vi "main 0.6.vi"() -> ()   [LabVIEW 2012]
uses:
  coherent/CH_LM/CH_LM Communication Mode.ctl
  ISEGNHQxxu/iseg NHQ VISA Control.ctl
  <vilib>/Utility/file.llb/Read From Spreadsheet File (DBL).vi
  <vilib>/Utility/file.llb/Write To Spreadsheet File (DBL).vi
  <vilib>/Analysis/1siggen.llb/Ramp Pattern by Samples.vi
  <vilib>/Analysis/NI_AALBase.lvlib
  coherent/CH_LM.lvlib
panel:
  out "laser power":sgl=6.5658234e-09 format="%^#_3e"
  out "Actual Voltage":dbl=-50.050000000000004 format="%.2f"
  out "Waveform Chart":dbl(graph)
  in  "Path":path=path "Y:/Ediff/data/2016/10/161018"
  in  "stop":bool
  out "Slide":dbl(slide)=0.999 scale=0.0..1.0
  in  "Tab Control":enum32{"live", "XY", "voltage scan", "settings"}(tab)
  in  "dark_load":bool
  in  "binning":dbl=4.0
  in  "exp time [s]":dbl=0.01
  in  "frames":i32=1000
  in  "avg[t] acc[f]":bool=TRUE
  in  "threshold":i32=110
  in  "dark?":bool=TRUE
  in  "dark":bool
  in  "snap":bool
  in  "count?":bool
  in  "save":bool
  in  "Nominal Voltage":sgl=50.0 max=4000 format="%.2f"
  in  "volt_set":bool
  in  "volt_threshold":sgl=2.0 max=4000 format="%.2f"
  in  "volt_timeout":u32=6000
  in  "move2com":bool
  in  "window2":dbl=10000.0 caption="+/- window" format="%#_6e"
  in  "steps2":u32=21 caption="steps"
  out "XY":dbl[][](graph)
  in  "meas_start_XY":bool
  in  "Axis2":string(combo)="4D Z"
  in  "Axis1":string(combo)="4D Z"
  in  "window1":dbl=10000.0 caption="+/- window" format="%#_6e"
  in  "steps1":u32=21 caption="steps"
  in  "meas_stop_XY":bool
  in  "showcom":bool
  out "XY Graph":cluster{"Ramp Pattern":dbl[], dbl[]}(graph)
  in  "voltage":string="225"
  in  "meas_stop_volt":bool
  in  "meas_start_vofalt":bool
  in  "head":string="PowerVoltScan1"
  in  "VISA ISEG":refnum<visa-resource-name>="COM6"
  in  "Channel (A)":enum16{"A", "B"}(ring)=enum."B"
  in  "IP address":string="172.24.192.135"
  out "error out":errorcluster
  out "coherent":errorcluster
  out "captured":dbl[][](graph)
  out "live":dbl[][](graph)
  in  "close":bool
  # "W"
  # "V"
  # "Axis2"
  # "Axis1"
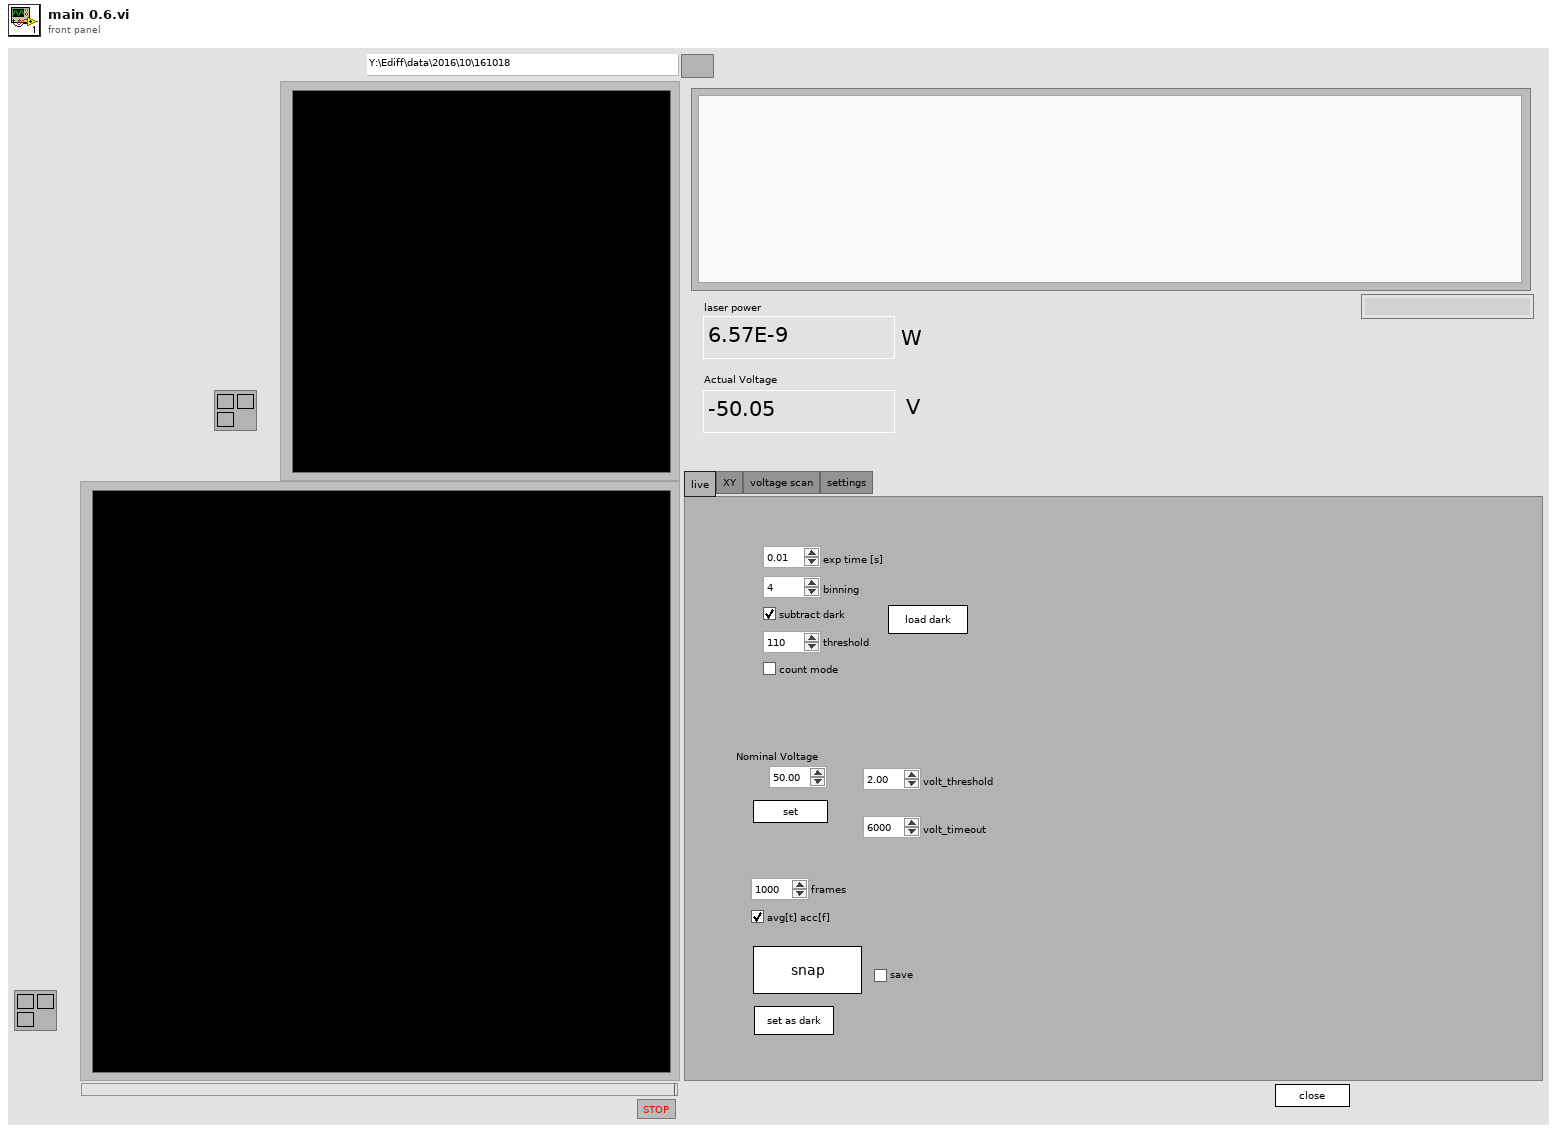
[diagram p1: front panel]
types:
  T1 = typedef "CH_LM.lvlib/CH_LM Communication Mode.ctl" = enum16{"None", "USB", "GPIB", "RS232"}
  T2 = cluster{"height":u32, "width":u32, "datatype":u32}
  T3 = typedef "iseg NHQ VISA Control.ctl" = cluster{"VISA Resource Name":refnum<visa-resource-name>, "FP Notation":bool, "Maximum Voltage":u32, "Maximum Current":u32}
  T4 = typedef "CH_LM.lvlib/CH_LM Streaming Data.ctl" = cluster{"Value":sgl, "Quad Distance":cluster{"X":sgl, "Y":sgl}, "Display Data":cluster{"Format ID":u8, "Scale ID":u8}, "Unit ID":u8, "Flags":u32, "Pulse Period":u32, "Sequence ID":u32, "Unit String":string}
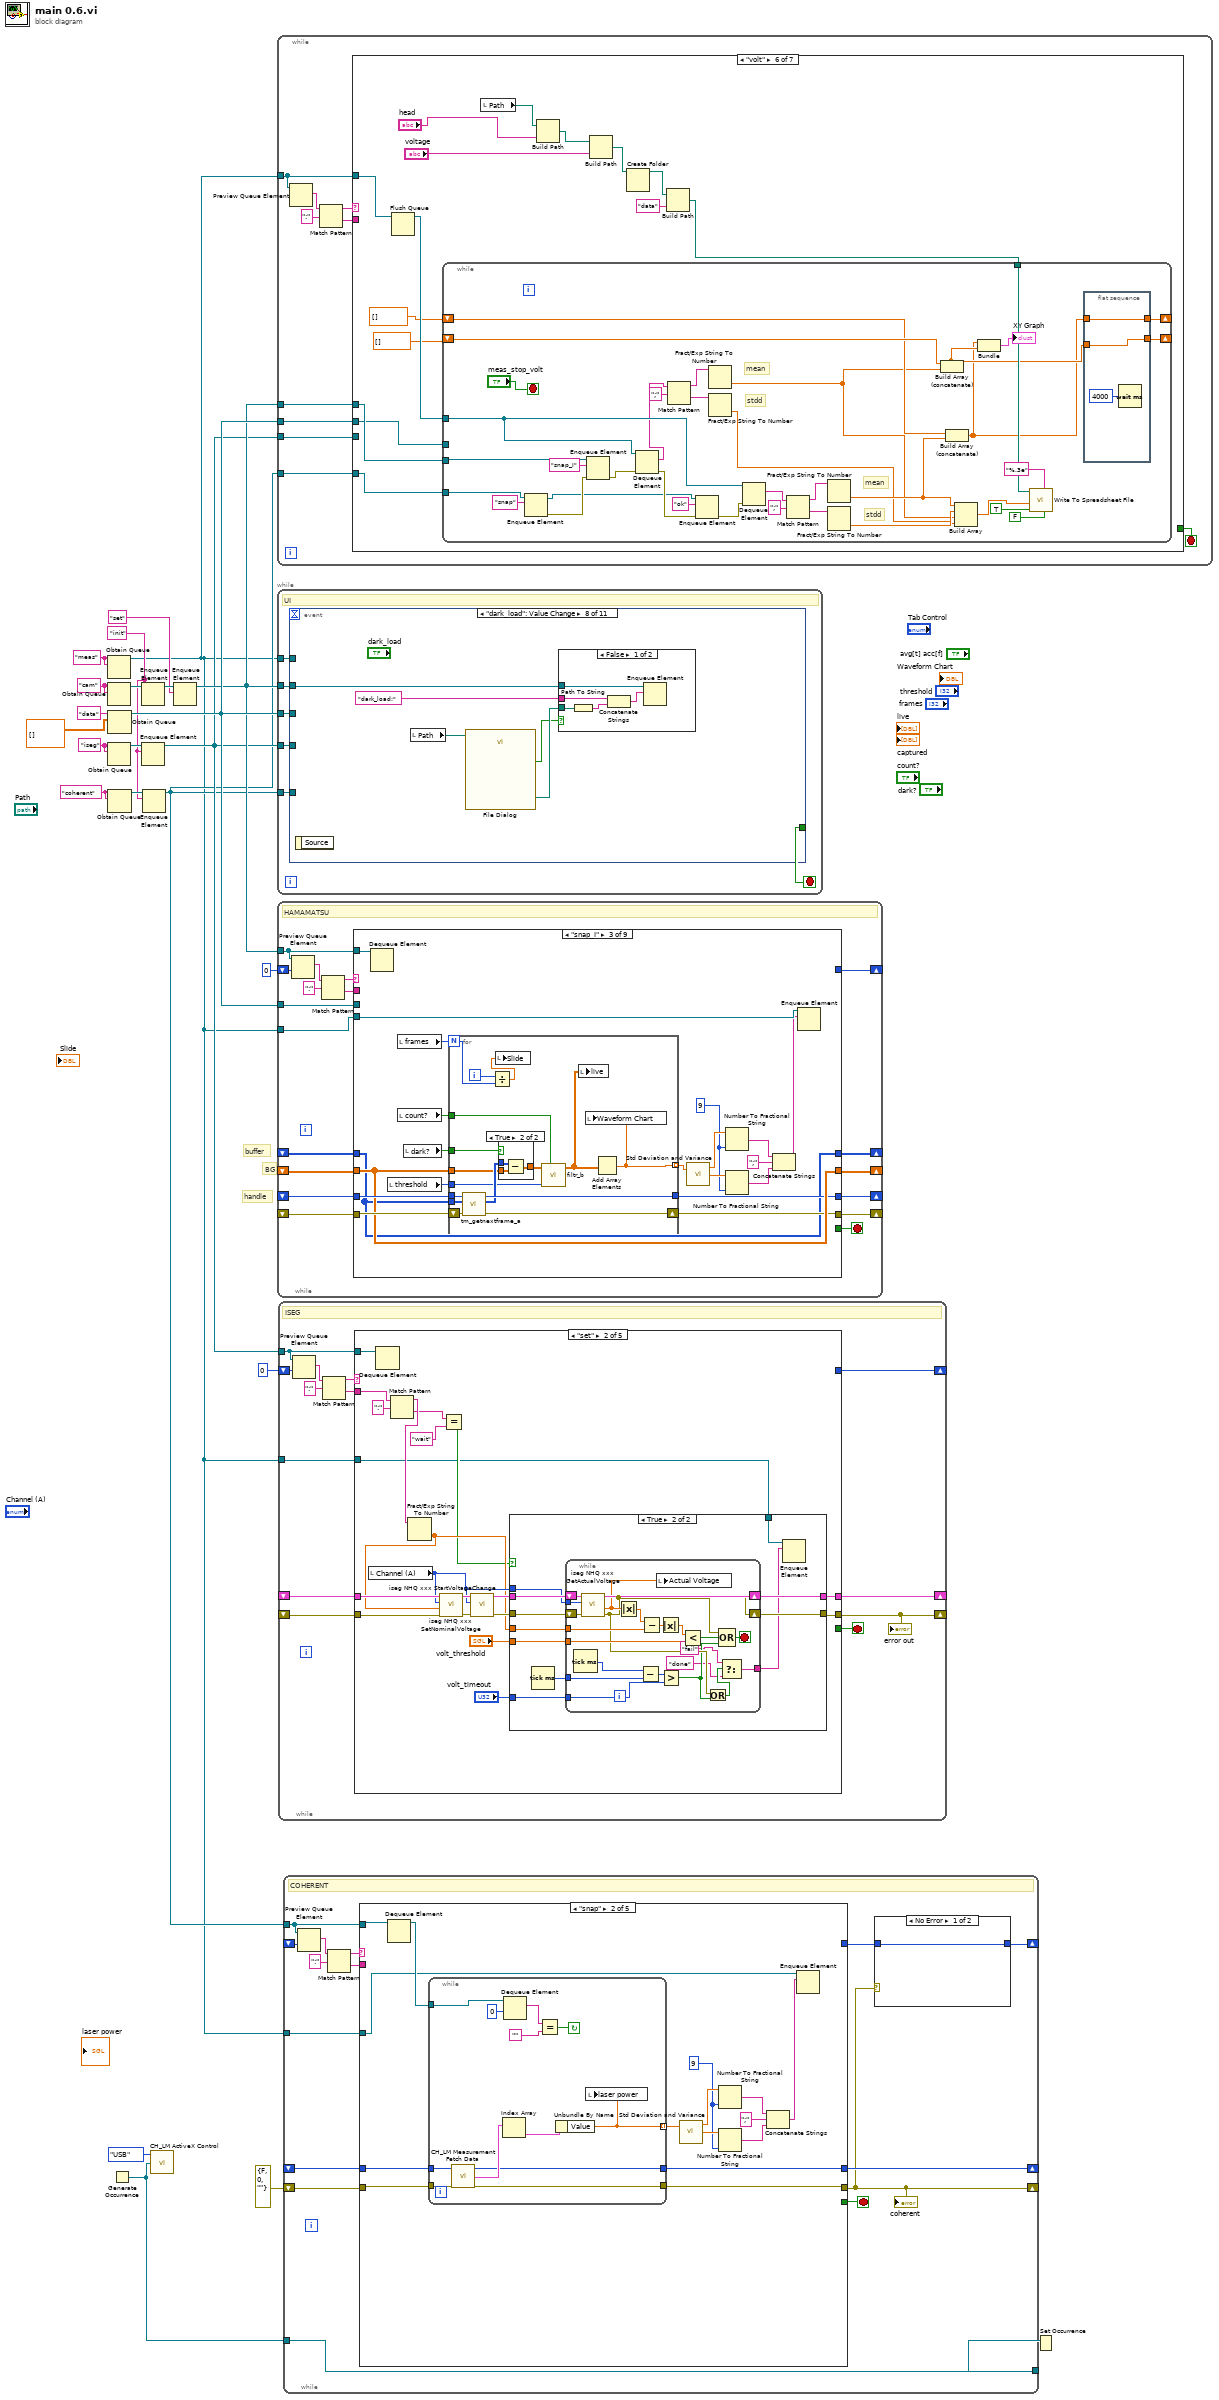
[diagram p0: block diagram]
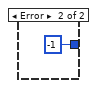
[diagram p2: hidden frame]
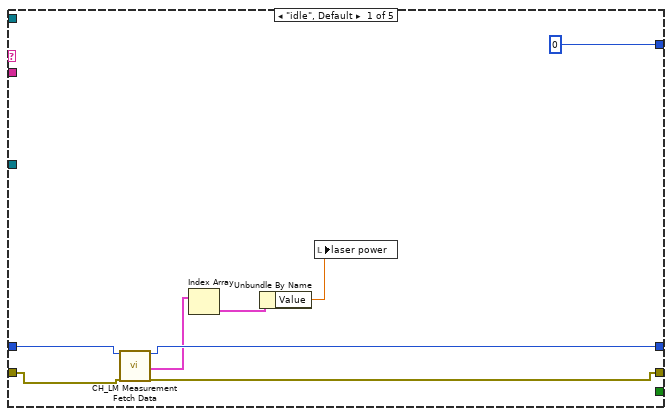
[diagram p3: hidden frame]
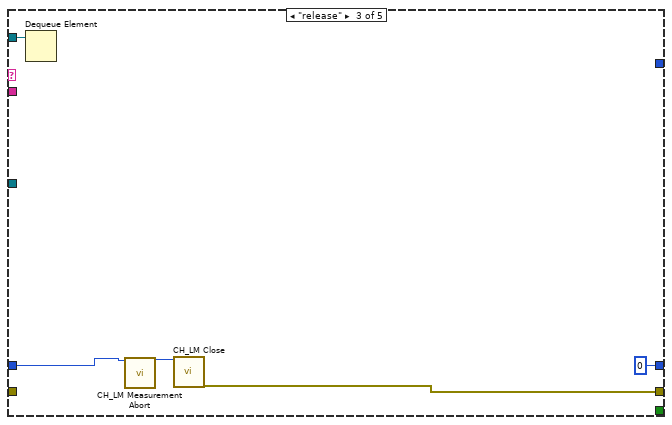
[diagram p4: hidden frame]
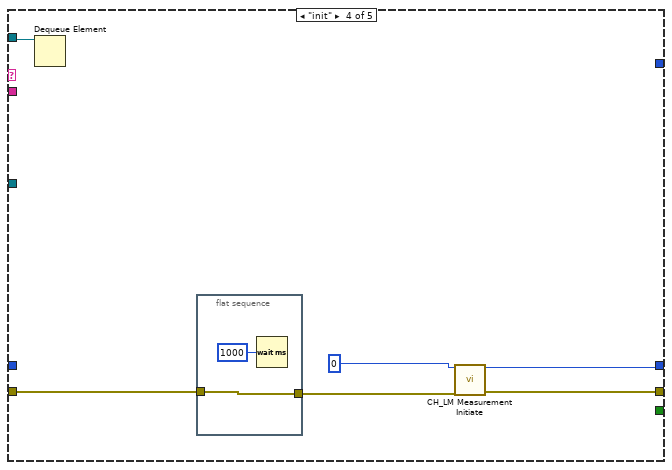
[diagram p5: hidden frame]
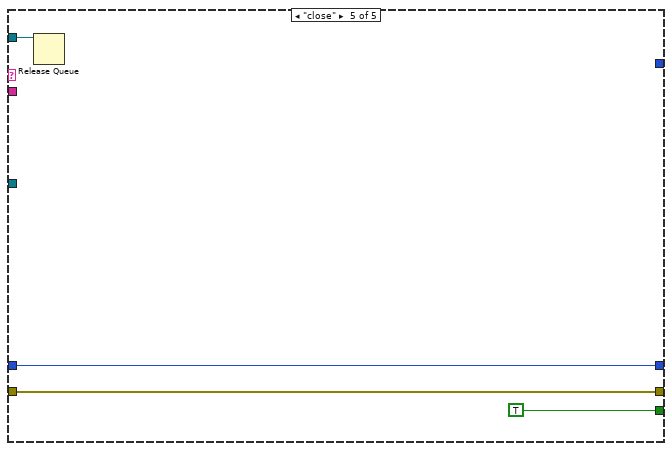
[diagram p6: hidden frame]
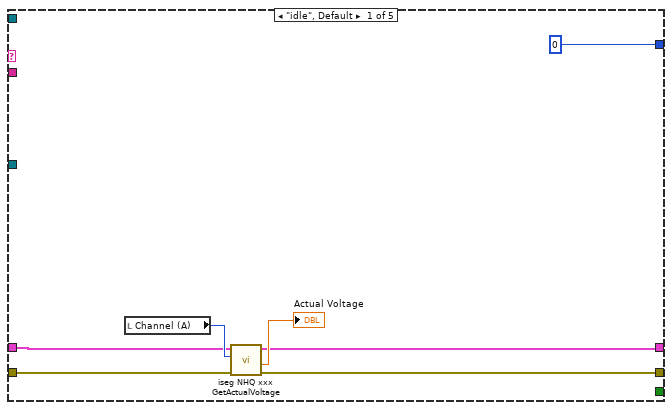
[diagram p7: hidden frame]
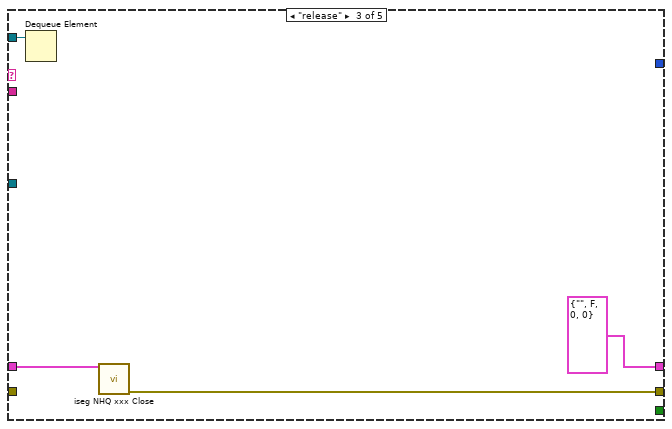
[diagram p9: hidden frame]
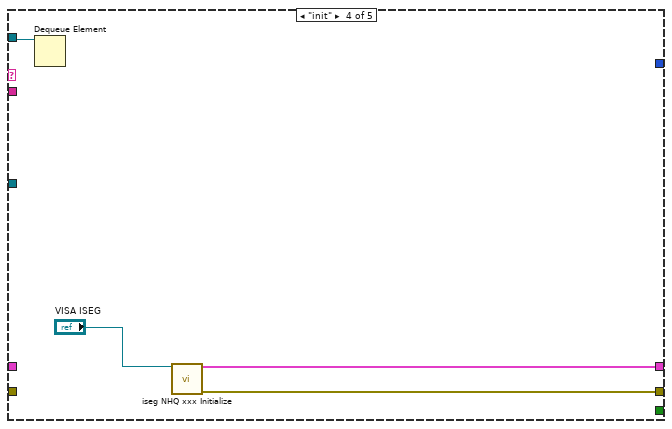
[diagram p10: hidden frame]
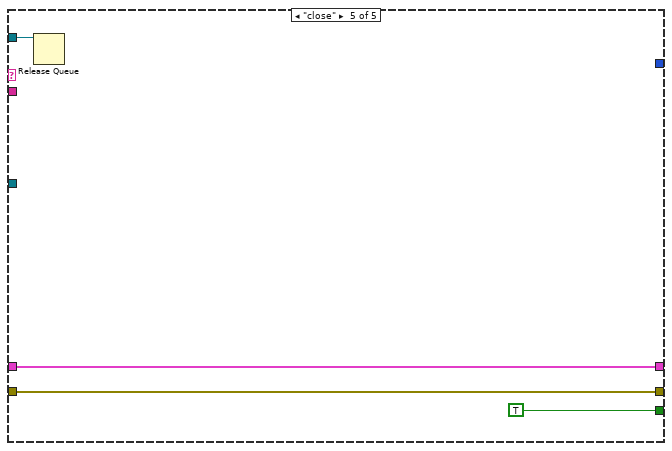
[diagram p11: hidden frame]
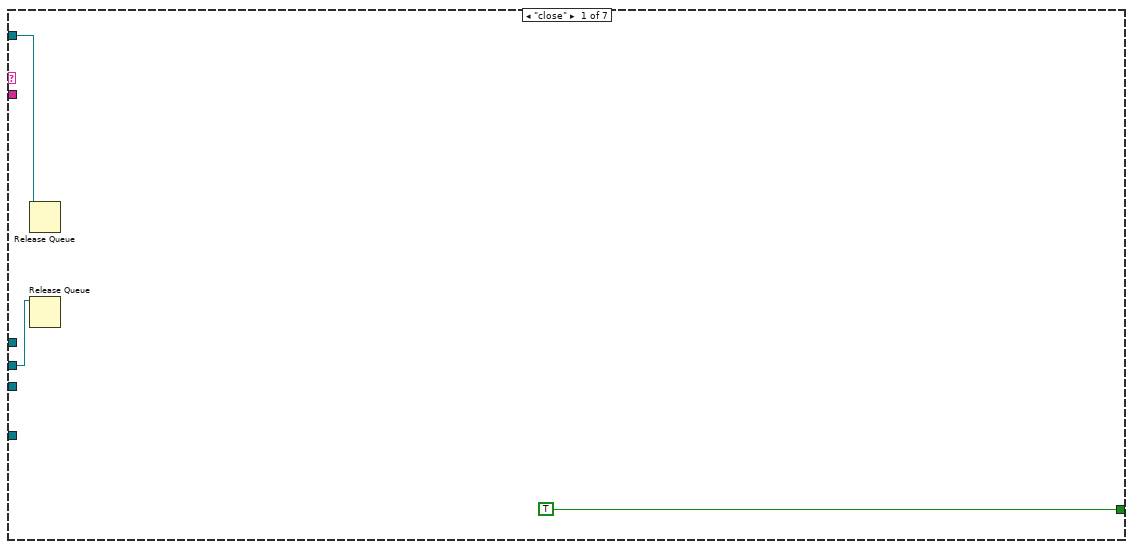
[diagram p12: hidden frame]
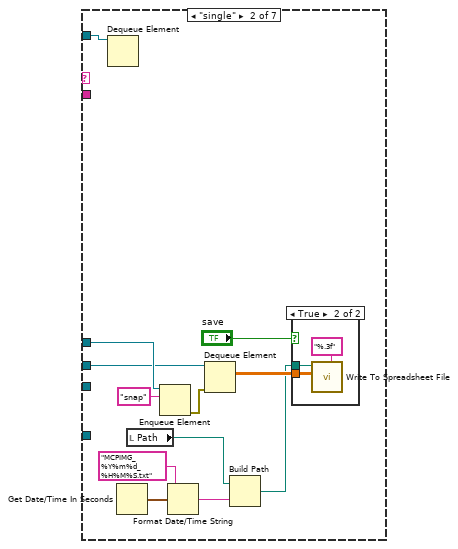
[diagram p13: hidden frame]
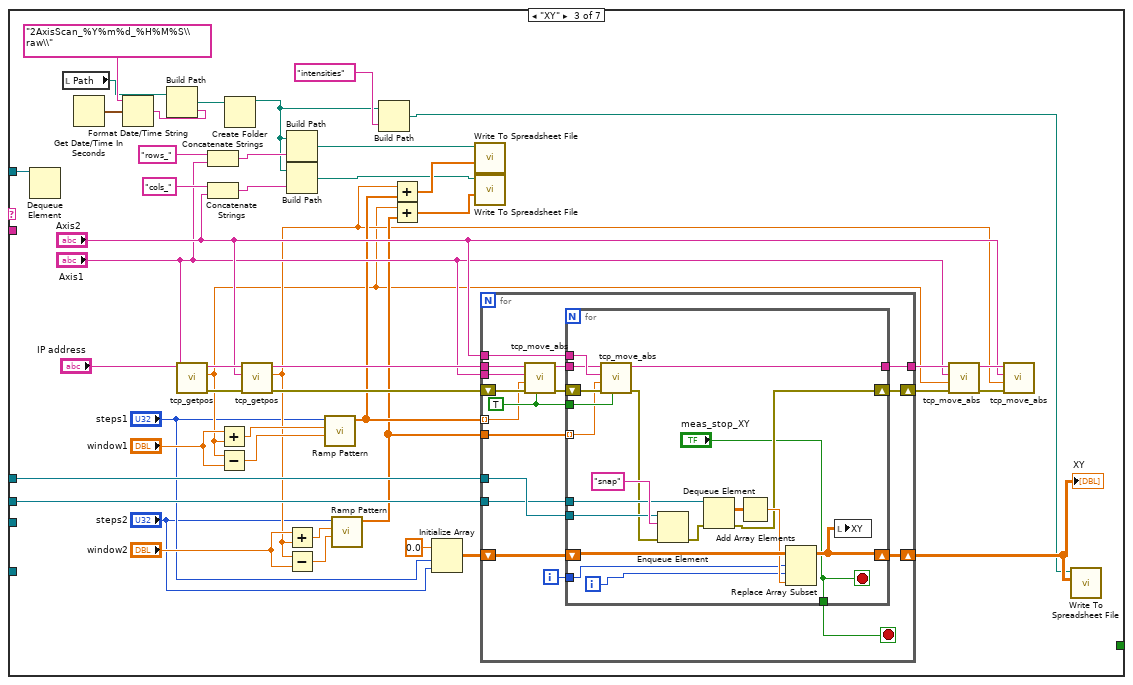
[diagram p15: hidden frame]
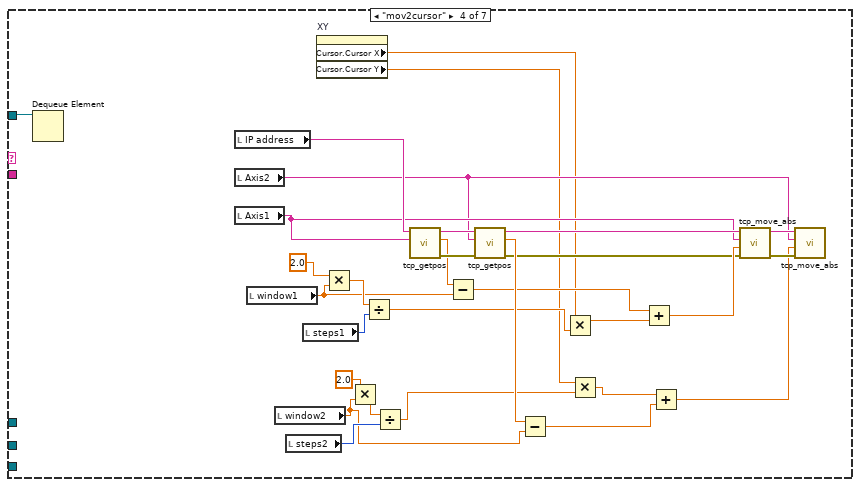
[diagram p16: hidden frame]
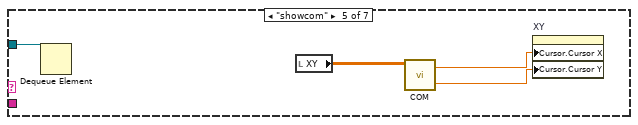
[diagram p17: hidden frame]
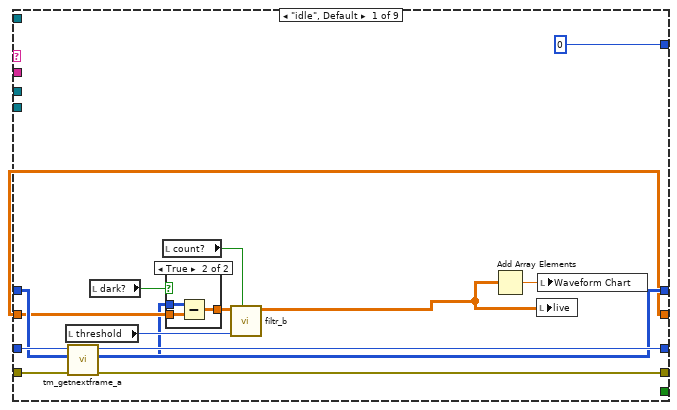
[diagram p19: hidden frame]
diagram:
  w8 = "coherent" ("name (unnamed)")
  w13 = "iseg" ("name (unnamed)")
  w7 = "init" ("element")
  w20 = "meas" ("name (unnamed)")
  w21 = "cam" ("name (unnamed)")
  # "BG"
  # "handle"
  # "buffer"
  n1 = Obtain Queue(name (unnamed)=w20, element data type=w20) -> (queue out=w1:refnum<queue>)  [unwired: 3 in, 2 out]
  n2 = Obtain Queue(name (unnamed)=w21, element data type=w21) -> (queue out=w23:refnum<queue>)  [unwired: 3 in, 2 out]
  n3 = Obtain Queue(name (unnamed)=w13, element data type=w13) -> (queue out=w12:refnum<queue>)  [unwired: 3 in, 2 out]
  n4 = Obtain Queue(name (unnamed)="data", element data type=dbl[][] []) -> (queue out=w16:refnum<queue>)  [unwired: 3 in, 2 out]
  n5 = Obtain Queue(name (unnamed)=w8, element data type=w8) -> (queue out=w9:refnum<queue>)  [unwired: 3 in, 2 out]
  n6 = Generate Occurrence() -> (w5:refnum<k4>)
  n7 = Enqueue Element(queue=w23, element=w7) -> (queue out=w19:refnum<queue>)  [unwired: 2 in, 2 out]
  n8 = Enqueue Element(queue=w12, element=w7) -> (queue out=w10:refnum<queue>)  [unwired: 2 in, 2 out]
  n9 = Enqueue Element(queue=w9, element=w7) -> (queue out=w3:refnum<queue>)  [unwired: 2 in, 2 out]
  n10 = call "CH_LM ActiveX Control.vi"("Communication Mode"=CH_LM_Communication_Mode."USB", "MonitorStop Occurrence"=w5) -> ()  [unwired: 3 in, 1 out]
  n11 = Enqueue Element(queue=w19, element="set") -> (queue out=w15:refnum<queue>)  [unwired: 2 in, 2 out]
  n12 = while {
    tunnel: w1 -> [w29]
    tunnel: w16 -> [w28]
    tunnel: w15 -> [w26]
    tunnel: w10 -> [w25]
    tunnel: w3 -> [w24]
    stop <- w27 stop-if-true
    n13 = Preview Queue Element(queue=w29) -> (element=w33:string)  [unwired: 2 in, 3 out]
    n14 = Match Pattern(string=w33, regular expression=":") -> (before substring=w31:string, after substring=w30:string)  [unwired: 1 in, 2 out]
    n15 = case shown="\"volt\"" w31 {
      tunnel: w30 -> [_ _ _ _ _ _ _]
      tunnel: w29 -> [w35 w48 w96 w162 w163 w181 _]
      tunnel: w28 -> [w36 w45 w92 _ _ w173 _]
      tunnel: [TRUE _ _ _ _ _ _] -> w27
      tunnel: w26 -> [_ w47 w93 _ _ w174 _]
      tunnel: w25 -> [_ _ _ _ _ _ _]
      tunnel: w24 -> [_ _ _ _ _ w175 _]
      frame "close" {
        n16 = Release Queue(queue=w35) -> ()  [unwired: 2 in, 3 out]
        n17 = Release Queue(queue=w36) -> ()  [unwired: 2 in, 3 out]
      }
      frame "single" {
        n18 = Dequeue Element(queue=w48) -> ()  [unwired: 2 in, 4 out]
        n19 = Get Date/Time In Seconds() -> (seconds since 1Jan1904=w41:timestamp)
        n20 = local read "Path"() -> (w37:path)
        n21 = Enqueue Element(queue=w47, element="snap") -> (error out=w44:errorcluster)  [unwired: 2 in, 2 out]
        n22 = Format Date/Time String(time format string (%c)="MCPIMG_%Y%m%d_%H%M%S.txt", seconds (now)=w41) -> (date/time string=w39:string)  [unwired: 1 in]
        n23 = Dequeue Element(queue=w45, error in (no error)=w44) -> (element=w43:dbl[][])  [unwired: 1 in, 3 out]
        n24 = Build Path(base path=w37, name or relative path=w39) -> (appended path=w38:path)
        n25 = case shown="True" "save" {
          tunnel: w43 -> [_ w51]
          tunnel: w38 -> [_ w49]
          frame False {
          }
          frame True {
            n26 = call-poly <vilib>:"Write To Spreadsheet File.vi"("format (%.3f)"="%.3f", "2D data"=w51, "file path (dialog if empty)"=w49) -> ()  [unwired: 5 in, 1 out]
          }
        }
      }
      frame "XY" {
        n27 = Dequeue Element(queue=w96) -> ()  [unwired: 2 in, 4 out]
        n28 = local read "Path"() -> (w87:path)
        n29 = Get Date/Time In Seconds() -> (seconds since 1Jan1904=w91:timestamp)
        n30 = Format Date/Time String(time format string (%c)="2AxisScan_%Y%m%d_%H%M%S\\raw\\", seconds (now)=w91) -> (date/time string=w55:string)  [unwired: 1 in]
        n31 = Build Path(base path=w87, name or relative path=w55) -> (appended path=w59:path)
        n32 = call "tcp_getpos.vi"("Axis"="Axis1", "IP address"="IP address") -> ("error out"=w88:errorcluster, "position"=w64:dbl, "IP address out"=w89:string)  [unwired: 7 in]
        n33 = Concatenate Strings("rows_" ("string"), "Axis1") -> (w56:string)
        n34 = Concatenate Strings("cols_" ("string"), "Axis2") -> (w86:string)
        n35 = Add(x="window1", y=w64) -> (x+y=w71:dbl)
        n36 = Subtract(x=w64, y="window1") -> (x-y=w70:dbl)
        n37 = Create Folder(path (use dialog)=w59) -> (created path=w54:path)  [unwired: 2 in, 2 out]
        n38 = call "tcp_getpos.vi"("error in (no error)"=w88, "Axis"="Axis2", "IP address"=w89) -> ("error out"=w81:errorcluster, "position"=w65:dbl, "IP address out"=w76:string)  [unwired: 6 in]
        n39 = Build Path(base path=w54, name or relative path=w56) -> (appended path=w53:path)
        n40 = Build Path(base path=w54, name or relative path=w86) -> (appended path=w52:path)
        n41 = Add(x="window2", y=w65) -> (x+y=w68:dbl)
        n42 = Subtract(x=w65, y="window2") -> (x-y=w69:dbl)
        n43 = call-poly <vilib>:"Ramp Pattern.vi"("start"=w70, "end"=w71, "samples"="steps1") -> ("Ramp Pattern"=w67:dbl[])  [unwired: 7 in, 1 out]
        n44 = call-poly <vilib>:"Ramp Pattern.vi"("start"=w69, "end"=w68, "samples"="steps2") -> ("Ramp Pattern"=w66:dbl[])  [unwired: 7 in, 1 out]
        n45 = Build Path(base path=w54, name or relative path="intensities") -> (appended path=w57:path)
        n46 = Add(x=w65, y=w67) -> (x+y=w63:dbl[])
        n47 = Add(x=w64, y=w66) -> (x+y=w62:dbl[])
        n48 = Initialize Array(0.0 ("element"), "steps1", "steps2") -> (w94:dbl[][])
        n49 = call-poly <vilib>:"Write To Spreadsheet File.vi"("1D data"=w63, "file path (dialog if empty)"=w53) -> ()  [unwired: 6 in, 1 out]
        n50 = call-poly <vilib>:"Write To Spreadsheet File.vi"("1D data"=w62, "file path (dialog if empty)"=w52) -> ()  [unwired: 6 in, 1 out]
        n51 = for {
          tunnel: "Axis1" -> [w113]
          tunnel: w93 -> [w112]
          tunnel: w92 -> [w111]
          tunnel: "Axis2" -> [w107]
          shift-right: [w106] -> w85
          shift-left: w94 -> [w110]
          shift-right: [w103] -> w82
          shift-left: w81 -> [w102]
          tunnel: [w100] -> w77
          tunnel: w76 -> [w99]
          tunnel: w67 -> [w97] mode=indexing
          tunnel: w66 -> [w98]
          i -> [w109]
          stop <- w101 stop-if-true
          w108 = TRUE ("wait4motiondone")
          n52 = call "tcp_move_abs.vi"("wait4motiondone"=w108, "error in (no error)"=w102, "destination nm/u°"=w97, "Axis"=w113, "IP address"=w99) -> ("error out"=w105:errorcluster, "IP address out"=w104:string)  [unwired: 4 in, 1 out]
          n53 = for {
            tunnel: w112 -> [w130]
            tunnel: w111 -> [w129]
            tunnel: w109 -> [w115]
            shift-right: [w120] -> w106
            shift-left: w110 -> [w128]
            tunnel: w108 -> [w124]
            tunnel: w107 -> [w123]
            tunnel: w104 -> [w121]
            shift-right: [w119] -> w103
            shift-left: w105 -> [w122]
            tunnel: ["meas_stop_XY"] -> w101
            tunnel: [w117] -> w100
            tunnel: w98 -> [w116] mode=indexing
            i -> [w114]
            stop <- "meas_stop_XY" stop-if-true
            n54 = call "tcp_move_abs.vi"("wait4motiondone"=w124, "error in (no error)"=w122, "destination nm/u°"=w116, "Axis"=w123, "IP address"=w121) -> ("error out"=w125:errorcluster, "IP address out"=w117:string)  [unwired: 4 in, 1 out]
            n55 = Enqueue Element(queue=w130, element="snap", error in (no error)=w125) -> (error out=w131:errorcluster)  [unwired: 1 in, 2 out]
            n56 = Dequeue Element(queue=w129, error in (no error)=w131) -> (element=w127:dbl[][], error out=w119:errorcluster)  [unwired: 1 in, 2 out]
            n57 = Add Array Elements(numeric array=w127) -> (sum=w126:dbl)
            n58 = Replace Array Subset(array=w128, new element=w126, index (row)=w115, index (col)=w114) -> (w120:dbl[][])
            n59 = local write "XY"(w120) -> ()
          }
        }
        "XY" <- w85
        n60 = call "tcp_move_abs.vi"("error in (no error)"=w82, "destination nm/u°"=w64, "Axis"="Axis1", "IP address"=w77) -> ("error out"=w84:errorcluster, "IP address out"=w83:string)  [unwired: 5 in, 1 out]
        n61 = call "tcp_move_abs.vi"("error in (no error)"=w84, "destination nm/u°"=w65, "Axis"="Axis2", "IP address"=w83) -> ()  [unwired: 5 in, 3 out]
        n62 = call-poly <vilib>:"Write To Spreadsheet File.vi"("2D data"=w85, "file path (dialog if empty)"=w57) -> ()  [unwired: 6 in, 1 out]
      }
      frame "mov2cursor" {
        n63 = Dequeue Element(queue=w162) -> ()  [unwired: 2 in, 4 out]
        n64 = local read "IP address"() -> (w157:string)
        n65 = local read "Axis2"() -> (w135:string)
        n66 = local read "Axis1"() -> (w136:string)
        n67 = local read "window1"() -> (w150:dbl)
        n68 = local read "window2"() -> (w149:dbl)
        n69 = local read "steps2"() -> (w155:u32)
        n70 = local read "steps1"() -> (w156:u32)
        n71 = property on="XY" class="IntGraph (strict)"() -> ("Cursor.Cursor X"=w134:dbl, "Cursor.Cursor Y"=w133:dbl)  [unwired: 2 in, 2 out]
        n72 = Multiply(x=2.0, y=w150) -> (x*y=w154:dbl)
        n73 = Multiply(x=2.0, y=w149) -> (x*y=w151:dbl)
        n74 = Divide(x=w154, y=w156) -> (x/y=w148:dbl)
        n75 = Divide(x=w151, y=w155) -> (x/y=w145:dbl)
        n76 = call "tcp_getpos.vi"("Axis"=w136, "IP address"=w157) -> ("error out"=w160:errorcluster, "position"=w158:dbl, "IP address out"=w161:string)  [unwired: 7 in]
        n77 = Subtract(x=w158, y=w150) -> (x-y=w146:dbl)
        n78 = call "tcp_getpos.vi"("error in (no error)"=w160, "Axis"=w135, "IP address"=w161) -> ("error out"=w138:errorcluster, "position"=w159:dbl, "IP address out"=w137:string)  [unwired: 6 in]
        n79 = Subtract(x=w159, y=w149) -> (x-y=w143:dbl)
        n80 = Multiply(x=w134, y=w148) -> (x*y=w147:dbl)
        n81 = Multiply(x=w133, y=w145) -> (x*y=w144:dbl)
        n82 = Add(x=w146, y=w147) -> (x+y=w140:dbl)
        n83 = Add(x=w144, y=w143) -> (x+y=w139:dbl)
        n84 = call "tcp_move_abs.vi"("error in (no error)"=w138, "destination nm/u°"=w140, "Axis"=w136, "IP address"=w137) -> ("error out"=w142:errorcluster, "IP address out"=w141:string)  [unwired: 5 in, 1 out]
        n85 = call "tcp_move_abs.vi"("error in (no error)"=w142, "destination nm/u°"=w139, "Axis"=w135, "IP address"=w141) -> ()  [unwired: 5 in, 3 out]
      }
      frame "showcom" {
        n86 = Dequeue Element(queue=w163) -> ()  [unwired: 2 in, 4 out]
        n87 = local read "XY"() -> (w166:dbl[][])
        n88 = call "COM.vi"("Array"=w166) -> ("Y out"=w164:dbl, "X out"=w165:dbl)  [unwired: 3 in]
        n89 = property on="XY" class="IntGraph (strict)"("Cursor.Cursor X"=w165, "Cursor.Cursor Y"=w164) -> ()  [unwired: 2 in, 2 out]
      }
      frame "volt" {
        n90 = Flush Queue(queue=w181) -> (queue out=w172:refnum<queue>)  [unwired: 1 in, 2 out]
        n91 = local read "Path"() -> (w180:path)
        n92 = Build Path(base path=w180, name or relative path="head") -> (appended path=w179:path)
        n93 = Build Path(base path=w179, name or relative path="voltage") -> (appended path=w177:path)
        n94 = Create Folder(path (use dialog)=w177) -> (created path=w167:path)  [unwired: 2 in, 2 out]
        n95 = Build Path(base path=w167, name or relative path="data") -> (appended path=w170:path)
        n96 = while {
          tunnel: w175 -> [w215]
          tunnel: w174 -> [w212]
          tunnel: w173 -> [_]
          tunnel: w172 -> [w188]
          tunnel: w170 -> [w205]
          shift-right: [w199] -> _
          shift-left: dbl[] [] -> [w204]
          shift-right: [w197] -> _
          shift-left: dbl[] [] -> [w203]
          stop <- "meas_stop_volt" stop-if-true
          # "stdd"
          # "mean"
          # "stdd"
          # "mean"
          n97 = Enqueue Element(queue=w215, element="snap") -> (queue out=w201:refnum<queue>, error out=w213:errorcluster)  [unwired: 2 in, 1 out]
          n98 = Enqueue Element(queue=w212, element="snap_I", error in (no error)=w213) -> (error out=w211:errorcluster)  [unwired: 1 in, 2 out]
          n99 = Dequeue Element(queue=w188, error in (no error)=w211) -> (element=w184:string, error out=w209:errorcluster)  [unwired: 1 in, 2 out]
          n100 = Match Pattern(string=w184, regular expression=";") -> (before substring=w187:string, after substring=w186:string)  [unwired: 1 in, 2 out]
          n101 = Enqueue Element(queue=w201, element="ok", error in (no error)=w209) -> (error out=w208:errorcluster)  [unwired: 1 in, 2 out]
          n102 = Fract/Exp String To Number(string=w187) -> (number=w183:dbl)  [unwired: 3 in, 1 out]
          n103 = Fract/Exp String To Number(string=w186) -> (number=w182:dbl)  [unwired: 3 in, 1 out]
          n104 = Dequeue Element(queue=w188, error in (no error)=w208) -> (element=w195:string)  [unwired: 1 in, 3 out]
          n105 = Match Pattern(string=w195, regular expression=";") -> (before substring=w193:string, after substring=w194:string)  [unwired: 1 in, 2 out]
          n106 = Fract/Exp String To Number(string=w193) -> (number=w192:dbl)  [unwired: 3 in, 1 out]
          n107 = Fract/Exp String To Number(string=w194) -> (number=w191:dbl)  [unwired: 3 in, 1 out]
          n108 = Build Array (concatenate)(w204, w183) -> (w200:dbl[])
          n109 = Build Array (concatenate)(w203, w192) -> (w198:dbl[])
          n110 = Build Array(w192, w191, w183, w182) -> (w190:dbl[])
          n111 = Bundle(w198, w200) -> (→"XY Graph":cluster{dbl[], dbl[]})  [unwired: 1 in]
          n112 = call-poly <vilib>:"Write To Spreadsheet File.vi"("transpose? (no:F)"=FALSE, "format (%.3f)"="%.3e", "append to file? (new file:F)"=TRUE, "1D data"=w190, "file path (dialog if empty)"=w205) -> ()  [unwired: 3 in, 1 out]
          n113 = flat-sequence {
            tunnel: w200 -> [w220]
            tunnel: [w220] -> w199
            tunnel: w198 -> [w219]
            tunnel: [w219] -> w197
            frame #0 {
              n114 = Wait (ms)(milliseconds to wait=u32 4000) -> ()  [unwired: 1 out]
            }
          }
        }
      }
      frame "idle", Default {
      }
    }
  }
  n115 = while {
    tunnel: w15 -> [w226]
    tunnel: w1 -> [w225]
    tunnel: w16 -> [w224]
    tunnel: w10 -> [w222]
    tunnel: w3 -> [w221]
    stop <- w223 stop-if-true
    # "UI"
    n116 = event shown="[7] \"dark_load\": Value Change" {
      selector: _ -> [_ _ _ _ _ _ _ _ _ _ _]
      dyn-events: _ -> [_ _ _ _ _ _ _ _ _ _ _]
      timeout: _ -> [_ _ _ _ _ _ _ _ _ _ _]
      tunnel: w226 -> [_ w235 w238 w240 _ _ _ w251 _ _ _]
      tunnel: w225 -> [_ w236 _ _ w241 w244 w245 _ w258 w260 _]
      tunnel: w224 -> [_ _ _ _ _ _ _ _ _ _ _]
      tunnel: [_ TRUE _ _ _ _ _ _ _ _ _] -> w223
      tunnel: w222 -> [_ w232 _ _ _ _ _ _ _ _ w265]
      tunnel: w221 -> [_ w229 _ _ _ _ _ _ _ _ _]
      event Timeout {
        n117 = event-data() -> ()  [unwired: 1 in, 1 out]
      }
      event "close": Value Change {
        w227 = "close" ("element")
        w228 = "release" ("element")
        n118 = event-data() -> ()  [unwired: 1 in, 1 out]
        n119 = Enqueue Element(queue=w229, element=w228) -> (queue out=w230:refnum<queue>)  [unwired: 2 in, 2 out]
        n120 = Enqueue Element(queue=w232, element=w228) -> (queue out=w231:refnum<queue>)  [unwired: 2 in, 2 out]
        n121 = Enqueue Element(queue=w235, element=w228) -> (queue out=w234:refnum<queue>)  [unwired: 2 in, 2 out]
        n122 = Enqueue Element(queue=w230, element=w227) -> ()  [unwired: 2 in, 3 out]
        n123 = Enqueue Element(queue=w231, element=w227) -> ()  [unwired: 2 in, 3 out]
        n124 = Enqueue Element(queue=w236, element=w227) -> ()  [unwired: 2 in, 3 out]
        n125 = Enqueue Element(queue=w234, element=w227) -> ()  [unwired: 2 in, 3 out]
      }
      event "dark": Value Change {
        n126 = event-data() -> ()  [unwired: 1 in, 1 out]
        n127 = Enqueue Element(queue=w238, element="dark") -> ()  [unwired: 2 in, 3 out]
      }
      event "binning", "exp time [s]": Value Change {
        n128 = event-data() -> ()  [unwired: 1 in, 1 out]
        n129 = Enqueue Element(queue=w240, element="set") -> ()  [unwired: 2 in, 3 out]
      }
      event "snap": Value Change {
        n130 = event-data() -> ()  [unwired: 1 in, 1 out]
        n131 = Enqueue Element(queue=w241, element="single") -> ()  [unwired: 2 in, 3 out]
      }
      event "meas_start_vofalt": Value Change {
        n132 = event-data() -> ()  [unwired: 1 in, 1 out]
        n133 = Enqueue Element(queue=w244, element="volt") -> ()  [unwired: 2 in, 3 out]
      }
      event "meas_start_XY": Value Change {
        n134 = event-data() -> ()  [unwired: 1 in, 1 out]
        n135 = Enqueue Element(queue=w245, element="XY") -> ()  [unwired: 2 in, 3 out]
      }
      event "dark_load": Value Change {
        n136 = event-data() -> ()  [unwired: 1 in, 1 out]
        n137 = local read "Path"() -> (w250:path)
        n138 = call "File Dialog"("start path"=w250) -> ("selected path"=w248:path, "cancelled"=w247:bool)  [unwired: 11 in, 2 out]
        n139 = case shown="False" w247 {
          tunnel: w251 -> [w256 _]
          tunnel: "dark_load:" ("element") -> [w254 _]
          tunnel: w248 -> [w252 _]
          frame False {
            n140 = Path To String(path=w252) -> (string=w253:string)
            n141 = Concatenate Strings(w254, w253) -> (w255:string)
            n142 = Enqueue Element(queue=w256, element=w255) -> ()  [unwired: 2 in, 3 out]
          }
          frame True {
          }
        }
      }
      event "move2com": Value Change {
        n143 = event-data() -> ()  [unwired: 1 in, 1 out]
        n144 = Enqueue Element(queue=w258, element="mov2cursor") -> ()  [unwired: 2 in, 3 out]
      }
      event "showcom": Value Change {
        n145 = event-data() -> ()  [unwired: 1 in, 1 out]
        n146 = Enqueue Element(queue=w260, element="showcom") -> ()  [unwired: 2 in, 3 out]
      }
      event "volt_set": Value Change {
        n147 = event-data() -> ()  [unwired: 1 in, 1 out]
        n148 = Number To Fractional String(number="Nominal Voltage") -> (F-format string=w261:string)  [unwired: 3 in]
        n149 = Concatenate Strings("set:" ("element"), w261) -> (w264:string)
        n150 = Enqueue Element(queue=w265, element=w264) -> ()  [unwired: 2 in, 3 out]
      }
    }
  }
  n151 = while {
    tunnel: w15 -> [w279]
    shift-right: [w277] -> _
    shift-left: _ -> [w276]
    shift-right: [w275] -> _
    shift-left: _ -> [w274]
    shift-right: [w273] -> _
    shift-left: _ -> [w272]
    shift-right: [w271] -> _
    shift-left: _ -> [w270]
    shift-right: [w268] -> _
    shift-left: 0 -> [w269]
    tunnel: w16 -> [w267]
    tunnel: w1 -> [w266]
    stop <- w278 stop-if-true
    # "HAMAMATSU"
    n152 = Preview Queue Element(queue=w279, timeout in ms (-1)=w269) -> (element=w283:string)  [unwired: 1 in, 3 out]
    n153 = Match Pattern(string=w283, regular expression=":") -> (before substring=w281:string, after substring=w280:string)  [unwired: 1 in, 2 out]
    n154 = case shown="\"snap_I\"" w281 {
      tunnel: w280 -> [_ _ _ _ w396 _ _ _ _]
      tunnel: w279 -> [_ w307 w350 w394 w401 w411 w412 w424 w453]
      tunnel: [_ _ _ _ _ _ _ _ TRUE] -> w278
      tunnel: [w292 w309 w362 w392 w398 w403 w417 w425 w448] -> w277
      tunnel: w276 -> [w294 w312 w364 w392 w398 w407 _ w447 w448]
      tunnel: [w293 w304 w361 w391 w399 u32 0 ("Handle out") w415 w426 w449] -> w275
      tunnel: w274 -> [w295 w310 w365 w391 w399 w408 _ w445 w449]
      tunnel: [w291 w311 w360 w393 w400 w409 w413 w427 w450] -> w273
      tunnel: w272 -> [w291 w311 w360 w393 w400 w409 w413 _ w450]
      tunnel: [w290 w308 w363 w390 w397 w410 w414 w428 w451] -> w271
      tunnel: w270 -> [w290 w308 w363 _ _ w410 w414 _ w451]
      tunnel: [0 _ _ _ _ _ _ _ _] -> w268
      tunnel: w267 -> [_ w303 _ _ _ _ _ _ _]
      tunnel: w266 -> [_ _ w352 _ _ _ _ _ _]
      frame "idle", Default {
        n155 = local read "threshold"() -> (w296:i32)
        n156 = call "tm_getnextframe_a.vi"("error in (no error)"=w294, "Buffer"=w291, "Handle in"=w295) -> ("error out"=w292:errorcluster, "Data"=w285:u16[][], "Handle out"=w293:u32)  [unwired: 6 in]
        n157 = local read "dark?"() -> (w297:bool)
        n158 = local read "count?"() -> (w287:bool)
        n159 = case shown="True" w297 {
          tunnel: [w298 w301] -> w288
          tunnel: w285 -> [w298 w300]
          tunnel: w290 -> [_ w299]
          frame False {
          }
          frame True {
            n160 = Subtract(x=w300, y=w299) -> (x-y=w301:dbl[][])
          }
        }
        n161 = call "filtr_b.vi"("count?"=w287, "threshold"=w296, "input array"=w288) -> ("output array"=w284:dbl[][])  [unwired: 8 in]
        n162 = Add Array Elements(numeric array=w284) -> (sum=w286:dbl)
        n163 = local write "live"(w284) -> ()
        n164 = local write "Waveform Chart"(w286) -> ()
      }
      frame "snap" {
        n165 = Dequeue Element(queue=w307) -> ()  [unwired: 2 in, 4 out]
        n166 = local read "avg[t] acc[f]"() -> (w306:bool)
        n167 = local read "threshold"() -> (w314:i32)
        n168 = local read "frames"() -> (w313:i32)
        n169 = local read "count?"() -> (w305:bool)
        n170 = local read "dark?"() -> (w315:bool)
        n171 = for {
          N: w313 -> [w321]
          tunnel: w315 -> [w335]
          tunnel: w311 -> [w333]
          tunnel: w310 -> [w334]
          tunnel: w314 -> [w327]
          tunnel: [w331] -> w304
          shift-right: [w330] -> w309
          shift-left: w312 -> [w332]
          tunnel: w308 -> [w326]
          shift-right: [w320] -> w302
          shift-left: w311 -> [w324]
          tunnel: w306 -> [w325]
          tunnel: w305 -> [w323]
          i -> [w322]
          stop <- "stop" stop-if-true
          n172 = call "tm_getnextframe_a.vi"("error in (no error)"=w332, "Buffer"=w333, "Handle in"=w334) -> ("error out"=w330:errorcluster, "Data"=w329:u16[][], "Handle out"=w331:u32)  [unwired: 6 in]
          n173 = Divide(x=w322, y=w321) -> (x/y=w317:dbl)
          n174 = case shown="True" w335 {
            tunnel: [w346 w349] -> w328
            tunnel: w329 -> [w346 w348]
            tunnel: w326 -> [_ w347]
            frame False {
            }
            frame True {
              n175 = Subtract(x=w348, y=w347) -> (x-y=w349:dbl[][])
            }
          }
          n176 = local write "Slide"(w317) -> ()
          n177 = call "filtr_b.vi"("count?"=w323, "threshold"=w327, "input array"=w328) -> ("output array"=w318:dbl[][])  [unwired: 8 in]
          n178 = Add Array Elements(numeric array=w318) -> (sum=w319:dbl)
          n179 = local write "live"(w318) -> ()
          n180 = local write "Waveform Chart"(w319) -> ()
          n181 = case shown="True" w325 {
            tunnel: w324 -> [w338 w345]
            tunnel: w318 -> [w337 w343]
            tunnel: [w336 w339] -> w320
            tunnel: w322 -> [_ w340]
            frame False {
              n182 = Add(x=w338, y=w337) -> (x+y=w336:dbl[][])
            }
            frame True {
              n183 = Multiply(x=w345, y=w340) -> (x*y=w344:dbl[][])
              n184 = Increment(x=w340) -> (x+1=w341:i32)
              n185 = Add(x=w344, y=w343) -> (x+y=w342:dbl[][])
              n186 = Divide(x=w342, y=w341) -> (x/y=w339:dbl[][])
            }
          }
          n187 = local write "captured"(w320) -> ()
        }
        n188 = local write "captured"(w302) -> ()
        n189 = Enqueue Element(queue=w303, element=w302) -> ()  [unwired: 2 in, 3 out]
      }
      frame "snap_I" {
        w355 = i16 9 ("precision (6)")
        n190 = Dequeue Element(queue=w350) -> ()  [unwired: 2 in, 4 out]
        n191 = local read "threshold"() -> (w368:i32)
        n192 = local read "frames"() -> (w367:i32)
        n193 = local read "count?"() -> (w366:bool)
        n194 = local read "dark?"() -> (w369:bool)
        n195 = for {
          N: w367 -> [w373]
          tunnel: w369 -> [w385]
          tunnel: w360 -> [w383]
          tunnel: w365 -> [w384]
          tunnel: w368 -> [w377]
          tunnel: [w381] -> w361
          shift-right: [w380] -> w362
          shift-left: w364 -> [w382]
          tunnel: w363 -> [w376]
          tunnel: w366 -> [w375]
          tunnel: [w370] -> w353 mode=indexing
          i -> [w374]
          n196 = call "tm_getnextframe_a.vi"("error in (no error)"=w382, "Buffer"=w383, "Handle in"=w384) -> ("error out"=w380:errorcluster, "Data"=w379:u16[][], "Handle out"=w381:u32)  [unwired: 6 in]
          n197 = Divide(x=w374, y=w373) -> (x/y=w372:dbl)
          n198 = local write "Slide"(w372) -> ()
          n199 = case shown="True" w385 {
            tunnel: [w386 w389] -> w378
            tunnel: w379 -> [w386 w388]
            tunnel: w376 -> [_ w387]
            frame False {
            }
            frame True {
              n200 = Subtract(x=w388, y=w387) -> (x-y=w389:dbl[][])
            }
          }
          n201 = call "filtr_b.vi"("count?"=w375, "threshold"=w377, "input array"=w378) -> ("output array"=w371:dbl[][])  [unwired: 8 in]
          n202 = local write "live"(w371) -> ()
          n203 = Add Array Elements(numeric array=w371) -> (sum=w370:dbl)
          n204 = local write "Waveform Chart"(w370) -> ()
        }
        n205 = call <vilib>:"Std Deviation and Variance.vi"("X"=w353) -> ("mean"=w359:dbl, "standard deviation"=w356:dbl)  [unwired: 1 in, 1 out]
        n206 = Number To Fractional String(number=w359, precision (6)=w355) -> (F-format string=w358:string)  [unwired: 2 in]
        n207 = Number To Fractional String(number=w356, precision (6)=w355) -> (F-format string=w354:string)  [unwired: 2 in]
        n208 = Concatenate Strings(w358, ";" ("string"), w354) -> (w351:string)
        n209 = Enqueue Element(queue=w352, element=w351) -> ()  [unwired: 2 in, 3 out]
      }
      frame "dark" {
        n210 = Dequeue Element(queue=w394) -> ()  [unwired: 2 in, 4 out]
        n211 = local read "captured"() -> (w390:dbl[][])
      }
      frame "dark_load" {
        n212 = Dequeue Element(queue=w401) -> ()  [unwired: 2 in, 4 out]
        n213 = String To Path(string=w396) -> (path=w395:path)
        n214 = call-poly <vilib>:"Read From Spreadsheet File.vi"("file path (dialog if empty)"=w395) -> ("all rows"=w397:dbl[][])  [unwired: 6 in, 4 out]
      }
      frame "release" {
        n215 = call "tm_stopcapture.vi"("error in (no error)"=w407, "Handle in"=w408) -> ("error out"=w405:errorcluster, "Handle out"=w406:u32)  [unwired: 8 in]
        n216 = Dequeue Element(queue=w411) -> ()  [unwired: 2 in, 4 out]
        n217 = call "tm_closecamera.vi"("error in (no error)"=w405, "Handle in"=w406) -> ("error out"=w404:errorcluster)  [unwired: 9 in]
        n218 = call "tm_deinitialize.vi"("error in (no error)"=w404) -> ("error out"=w403:errorcluster)  [unwired: 10 in]
      }
      frame "init" {
        n219 = Dequeue Element(queue=w412) -> ()  [unwired: 2 in, 4 out]
        n220 = call "tm_initialize.vi"() -> ("error out"=w418:errorcluster)  [unwired: 8 in, 3 out]
        n221 = call "tm_opencamera.vi"("error in (no error)"=w418, "Camera Index"=u32 0) -> ("error out"=w417:errorcluster, "Handle out"=w415:u32)  [unwired: 7 in, 1 out]
      }
      frame "set" {
        w433 = 1 items=["Snap", "Sequence"] ("Capture mode")
        w437 = u32 4215968 items=["BINNING"=4215968, "BITS PER CHANNEL"=2, "ACTIVE VIEW INDEX"=3, "CCD MODE"=4, "SENSOR MODE"=5, "READOUT MODE"=6, "EXPOSURE TIME"=7, "CONTRAST GAIN"=8, "CONTRAST OFFSET"=9, "LIGHT MODE"=10, "SENSITIVITY"=11, "WHITE BALANCE"=12, "PHOTON IMAGING MODE"=13, "HIGH DYNAMIC RANGE MODE"=14, "TRIGGER SOURCE"=15, "TRIGGER ACTIVE"=16, "TRIGGER MODE"=17, "TRIGGER POLARITY"=18, "TRIGGER GLOBAL EXPOSURE"=19, "FIRST TRIGGER BEHAVIOR"=20, "TRIGGER TIMES"=21, "OUTPUT TRIGGER POLARITY"=22, "OUTPUT TRIGGER DELAY"=23, "OUTPUT TRIGGER PERIOD"=24, "TEMPERATURE"=25, "TEMPERATURE TARGET"=26, "SENSOR COOLER FAN"=27, "MECHANICAL SHUTTER"=28, "BACK FOCUS POSITION"=29, "FRAMEBUNDLE MODE"=30, "FRAMEBUNDLE NUMBER"=31, "LINEBUNDLE HEIGHT"=32, "TRIGGER CONNECTOR"=33, "IMAGE PIXEL TYPE"=34, "OUTPUT TRIGGER KIND"=35, "READOUT DIRECTION"=36, "CHANNEL SYNC"=37] ("Parameter")
        w441 = u32 7 items=["BINNING"=4215968, "BITS PER CHANNEL"=2, "ACTIVE VIEW INDEX"=3, "CCD MODE"=4, "SENSOR MODE"=5, "READOUT MODE"=6, "EXPOSURE TIME"=7, "CONTRAST GAIN"=8, "CONTRAST OFFSET"=9, "LIGHT MODE"=10, "SENSITIVITY"=11, "WHITE BALANCE"=12, "PHOTON IMAGING MODE"=13, "HIGH DYNAMIC RANGE MODE"=14, "TRIGGER SOURCE"=15, "TRIGGER ACTIVE"=16, "TRIGGER MODE"=17, "TRIGGER POLARITY"=18, "TRIGGER GLOBAL EXPOSURE"=19, "FIRST TRIGGER BEHAVIOR"=20, "TRIGGER TIMES"=21, "OUTPUT TRIGGER POLARITY"=22, "OUTPUT TRIGGER DELAY"=23, "OUTPUT TRIGGER PERIOD"=24, "TEMPERATURE"=25, "TEMPERATURE TARGET"=26, "SENSOR COOLER FAN"=27, "MECHANICAL SHUTTER"=28, "BACK FOCUS POSITION"=29, "FRAMEBUNDLE MODE"=30, "FRAMEBUNDLE NUMBER"=31, "LINEBUNDLE HEIGHT"=32, "TRIGGER CONNECTOR"=33, "IMAGE PIXEL TYPE"=34, "OUTPUT TRIGGER KIND"=35, "READOUT DIRECTION"=36, "CHANNEL SYNC"=37] ("Parameter")
        n222 = Dequeue Element(queue=w424) -> ()  [unwired: 2 in, 4 out]
        n223 = call "tm_stopcapture.vi"("error in (no error)"=w447, "Handle in"=w445) -> ("error out"=w446:errorcluster, "Handle out"=w444:u32)  [unwired: 8 in]
        n224 = call "tm_unpreparecapture.vi"("error in (no error)"=w446, "Handle in"=w444) -> ("error out"=w443:errorcluster, "Handle out"=w442:u32)  [unwired: 8 in]
        n225 = call "tm_setparameter.vi"("error in (no error)"=w443, "Value in"="exp time [s]", "Parameter"=w441, "Handle in"=w442) -> ("error out"=w438:errorcluster, "Handle out"=w439:u32)  [unwired: 6 in]
        n226 = call "tm_setparameter.vi"("error in (no error)"=w438, "Value in"="binning", "Parameter"=w437, "Handle in"=w439) -> ("error out"=w434:errorcluster, "Handle out"=w435:u32)  [unwired: 6 in]
        n227 = call "tm_preparecapture.vi"("error in (no error)"=w434, "Frames"=1, "Capture mode"=w433, "Handle in"=w435) -> ("error out"=w430:errorcluster, "Buffer Info"=w429:T2, "Handle out"=w431:u32)  [unwired: 4 in, 1 out]
        n228 = Unbundle(w429) -> ("height"=w422:u32, "width"=w423:u32)  [unwired: 1 out]
        n229 = call "tm_startcapture_b.vi"("error in (no error)"=w430, "Handle in"=w431) -> ("error out"=w425:errorcluster, "Handle out"=w426:u32)  [unwired: 8 in]
        n230 = property on="live" class="IntGraph (strict)"("XScale.Minimum"=0.0 ("X Scale.Range:Minimum"), "XScale.Maximum"=w422, "YScale.Minimum"=0.0 ("Y Scale.Range:Minimum"), "YScale.Maximum"=w423) -> ()  [unwired: 2 in, 2 out]
        n231 = Initialize Array(u16 0 ("element"), w422, w423) -> (w427:u16[][])
        n232 = To Double Precision Float(number=w427) -> (double precision float=w428:dbl[][])
      }
      frame "close" {
        n233 = Release Queue(queue=w453) -> ()  [unwired: 2 in, 3 out]
      }
    }
  }
  n234 = while {
    tunnel: w10 -> [w462]
    shift-right: [w460] -> _
    shift-left: _ -> [w459]
    shift-right: [w457] -> _
    shift-left: 0 -> [w458]
    shift-right: [w456] -> _
    shift-left: _ -> [w455]
    tunnel: w1 -> [w454]
    stop <- w461 stop-if-true
    # "ISEG"
    n235 = Preview Queue Element(queue=w462, timeout in ms (-1)=w458) -> (element=w466:string)  [unwired: 1 in, 3 out]
    n236 = Match Pattern(string=w466, regular expression=":") -> (before substring=w464:string, after substring=w463:string)  [unwired: 1 in, 2 out]
    n237 = case shown="\"set\"" w464 {
      tunnel: w463 -> [_ w479 _ _ _]
      tunnel: w462 -> [_ w491 w532 w536 w540]
      tunnel: [_ _ _ _ TRUE] -> w461
      tunnel: [w467 w485 w530 w535 w537] -> w460
      tunnel: w459 -> [w469 w489 _ _ w537]
      tunnel: [0 _ _ _ _] -> w457
      tunnel: [w468 w486 T3 {"VISA Resource Name"="", "FP Notation"=FALSE, "Maximum Voltage"=0, "Maximum Current"=0} ("VISA Session Out") w533 w538] -> w456
      tunnel: w455 -> [w470 w490 w531 _ w538]
      tunnel: w454 -> [_ w474 _ _ _]
      frame "idle", Default {
        n238 = local read "Channel (A)"() -> (w472:enum16{"A", "B"})
        n239 = call "iseg NHQ xxx GetActualVoltage.vi"("error in (no error)"=w469, "Channel (A)"=w472, "VISA Session"=w470) -> ("error out"=w467:errorcluster, "Voltage"=→"Actual Voltage":dbl, "VISA Session Out"=w468:T3)  [unwired: 5 in, 1 out]
      }
      frame "set" {
        n240 = local read "Channel (A)"() -> (w482:enum16{"A", "B"})
        n241 = Dequeue Element(queue=w491) -> ()  [unwired: 2 in, 4 out]
        n242 = Match Pattern(string=w479, regular expression=":") -> (before substring=w478:string, after substring=w477:string)  [unwired: 1 in, 2 out]
        n243 = Fract/Exp String To Number(string=w478) -> (number=w481:dbl)  [unwired: 3 in, 1 out]
        n244 = call "iseg NHQ xxx SetNominalVoltage.vi"("error in (no error)"=w489, "Voltage (0 V)"=w481, "Channel (A)"=w482, "VISA Session"=w490) -> ("error out"=w492:errorcluster, "VISA Session Out"=w493:T3)  [unwired: 6 in]
        n245 = Equal?(x=w477, y="wait") -> (x = y?=w475:bool)
        n246 = call "iseg NHQ xxx StartVoltageChange.vi"("error in (no error)"=w492, "Channel (A)"=w482, "VISA Session"=w493) -> ("error out"=w487:errorcluster, "VISA Session Out"=w488:T3)  [unwired: 6 in, 1 out]
        n247 = case shown="True" w475 {
          tunnel: [w495 w505] -> w486
          tunnel: [w494 w497] -> w485
          tunnel: w488 -> [w495 w504]
          tunnel: w487 -> [w494 w503]
          tunnel: w481 -> [_ w502]
          tunnel: "volt_threshold" -> [_ w501]
          tunnel: "volt_timeout" -> [_ w500]
          tunnel: w482 -> [_ w499]
          tunnel: w474 -> [_ w498]
          frame False {
          }
          frame True {
            n248 = Tick Count (ms)() -> (millisecond timer value=w506:u32)
            n249 = while {
              shift-right: [w526] -> w505
              shift-left: w504 -> [w528]
              shift-right: [w512] -> w497
              shift-left: w503 -> [w527]
              tunnel: w499 -> [w525]
              tunnel: w501 -> [w522]
              tunnel: w506 -> [w520]
              tunnel: w500 -> [w518]
              tunnel: w502 -> [w517]
              tunnel: [w507] -> w496
              stop <- w513 stop-if-true
              n250 = Tick Count (ms)() -> (millisecond timer value=w521:u32)
              n251 = call "iseg NHQ xxx GetActualVoltage.vi"("error in (no error)"=w527, "Channel (A)"=w525, "VISA Session"=w528) -> ("error out"=w512:errorcluster, "Voltage"=w515:dbl, "VISA Session Out"=w526:T3)  [unwired: 5 in, 1 out]
              n252 = Absolute Value(x=w515) -> (abs(x)=w516:dbl)
              n253 = Subtract(x=w521, y=w520) -> (x-y=w519:u32)
              n254 = Subtract(x=w516, y=w517) -> (x-y=w524:dbl)
              n255 = local write "Actual Voltage"(w515) -> ()
              n256 = Absolute Value(x=w524) -> (abs(x)=w523:dbl)
              n257 = Greater?(x=w519, y=w518) -> (0:w511:bool)
              n258 = Less?(x=w523, y=w522) -> (x < y?=w514:bool)
              n259 = Or(x=w512, y=w511) -> (x .or. y?=w510:bool)
              n260 = Compound Arithmetic op=OR(w512, w514, w511) -> (w513:bool)
              n261 = Select(t="fail" ("element"), s=w510, f="done" ("element")) -> (s? t:f=w507:string)
            }
            n262 = Enqueue Element(queue=w498, element=w496) -> ()  [unwired: 2 in, 3 out]
          }
        }
      }
      frame "release" {
        n263 = Dequeue Element(queue=w532) -> ()  [unwired: 2 in, 4 out]
        n264 = call "iseg NHQ xxx Close.vi"("VISA session"=w531) -> ("error out"=w530:errorcluster)  [unwired: 14 in]
      }
      frame "init" {
        n265 = Dequeue Element(queue=w536) -> ()  [unwired: 2 in, 4 out]
        n266 = call "iseg NHQ xxx Initialize.vi"("VISA resource name"="VISA ISEG") -> ("VISA Session Out"=w533:T3, "error out"=w535:errorcluster)  [unwired: 13 in]
      }
      frame "close" {
        n267 = Release Queue(queue=w540) -> ()  [unwired: 2 in, 3 out]
      }
    }
    "error out" <- w460
  }
  n268 = while {
    tunnel: w3 -> [w551]
    shift-right: [w541] -> _
    shift-left: errorcluster {"status"=FALSE, "code"=0, "source"=""} ("error constant") -> [w549]
    shift-right: [w543] -> _
    shift-left: _ -> [w548]
    shift-right: [w547] -> _
    shift-left: _ -> [w546]
    tunnel: w1 -> [w545]
    tunnel: w5 -> [w544]
    tunnel: [w544] -> w4
    stop <- w550 stop-if-true
    # "COHERENT"
    n269 = Preview Queue Element(queue=w551, timeout in ms (-1)=w548) -> (element=w555:string)  [unwired: 1 in, 3 out]
    n270 = Match Pattern(string=w555, regular expression=":") -> (before substring=w553:string, after substring=w552:string)  [unwired: 1 in, 2 out]
    n271 = case shown="\"snap\"" w553 {
      tunnel: w552 -> [_ _ _ _ _]
      tunnel: w551 -> [_ w580 w597 w603 w609]
      tunnel: [_ _ _ _ TRUE] -> w550
      tunnel: [w561 w572 w595 w600 w606] -> w541
      tunnel: w549 -> [w563 w577 _ w599 w606]
      tunnel: [0 _ _ _ _] -> w542
      tunnel: [w562 w573 0 ("Meter Index") w601 w607] -> w547
      tunnel: w546 -> [w564 w578 w593 _ w607]
      tunnel: w545 -> [_ w576 _ _ _]
      frame "idle", Default {
        n272 = call "CH_LM Measurement Fetch Data.vi"("Meter Index"=w564, "error in (no error)"=w563) -> ("Meter Index"=w562:i32, "Data Array"=w560:T4[], "error out"=w561:errorcluster)  [unwired: 13 in, 2 out]
        n273 = Index Array(array=w560) -> (element=w559:T4)  [unwired: 1 in]
        n274 = Unbundle By Name(w559) -> ("Value"=w558:sgl)
        n275 = local write "laser power"(w558) -> ()
      }
      frame "snap" {
        w568 = i16 9 ("precision (6)")
        n276 = Dequeue Element(queue=w580) -> (queue out=w579:refnum<queue>)  [unwired: 2 in, 3 out]
        n277 = while {
          tunnel: w579 -> [w589]
          tunnel: w578 -> [w586]
          tunnel: w577 -> [w585]
          tunnel: [w581] -> w575 mode=indexing
          tunnel: [w584] -> w573
          tunnel: [w583] -> w572
          stop <- w590 continue-if-true
          n278 = call "CH_LM Measurement Fetch Data.vi"("Meter Index"=w586, "error in (no error)"=w585) -> ("Meter Index"=w584:i32, "Data Array"=w588:T4[], "error out"=w583:errorcluster)  [unwired: 13 in, 2 out]
          n279 = Index Array(array=w588) -> (element=w587:T4)  [unwired: 1 in]
          n280 = Dequeue Element(queue=w589, timeout in ms (-1)=0) -> (element=w592:string)  [unwired: 1 in, 3 out]
          n281 = Equal?(x=w592, y="") -> (x = y?=w590:bool)
          n282 = Unbundle By Name(w587) -> ("Value"=w581:sgl)
          n283 = local write "laser power"(w581) -> ()
        }
        n284 = call <vilib>:"Std Deviation and Variance.vi"("X"=w575) -> ("mean"=w574:dbl, "standard deviation"=w569:dbl)  [unwired: 1 in, 1 out]
        n285 = Number To Fractional String(number=w574, precision (6)=w568) -> (F-format string=w571:string)  [unwired: 2 in]
        n286 = Number To Fractional String(number=w569, precision (6)=w568) -> (F-format string=w567:string)  [unwired: 2 in]
        n287 = Concatenate Strings(w571, ";" ("string"), w567) -> (w566:string)
        n288 = Enqueue Element(queue=w576, element=w566) -> ()  [unwired: 2 in, 3 out]
      }
      frame "release" {
        n289 = Dequeue Element(queue=w597) -> ()  [unwired: 2 in, 4 out]
        n290 = call "CH_LM Measurement Abort.vi"("Meter Index"=w593) -> ("Meter Index"=w594:i32)  [unwired: 16 in, 2 out]
        n291 = call "CH_LM Close.vi"("Meter Index"=w594) -> ("error out"=w595:errorcluster)  [unwired: 16 in, 2 out]
      }
      frame "init" {
        n292 = Dequeue Element(queue=w603) -> ()  [unwired: 2 in, 4 out]
        n293 = flat-sequence {
          tunnel: w599 -> [w605]
          tunnel: [w605] -> w598
          frame #0 {
            n294 = Wait (ms)(milliseconds to wait=u32 1000) -> ()  [unwired: 1 out]
          }
        }
        n295 = call "CH_LM Measurement Initiate.vi"("Meter Index"=0, "error in (no error)"=w598) -> ("Meter Index"=w601:i32, "error out"=w600:errorcluster)  [unwired: 15 in, 1 out]
      }
      frame "close" {
        n296 = Release Queue(queue=w609) -> ()  [unwired: 2 in, 3 out]
      }
    }
    "coherent" <- w541
    n297 = case shown="No Error" w541 {
      tunnel: [w556 -1] -> w543
      tunnel: w542 -> [w556 _]
      frame No Error {
      }
      frame Error {
      }
    }
  }
  n298 = Set Occurrence(w4) -> ()
